vi "niScope Multi Fetch WDT_noERROR.vi"(6 "numSamples":i32=-1, 7 "timestamp Type":T1=1 caption="timestamp type" items=["relative", "absolute"], 8 "error in":errorcluster, 9 "timeout":dbl=5.0 format="%.2f", 10 "channels":string="0", 11 "instrument handle":refnum<k15>) -> (0 "error out":errorcluster, 1 "wfm":waveform(dbl)[](array[waveform]), 2 "wfm info":T2(array[cluster]) {"reserved2" format="%.2f"; "reserved1" format="%.2f"; "offset" format="%^.3e"; "gain" format="%^.3e"; "xIncrement" format="%^.3e"; "relativeInitialX" format="%^.3e"; "absoluteInitialX" format="%^.3e"}, 3 "instrument handle out":refnum<k15>)   [LabVIEW 2010]
uses:
  <instrlib>/niScope/Controls/niScope timestamp type.ctl
  niScope_32.dll
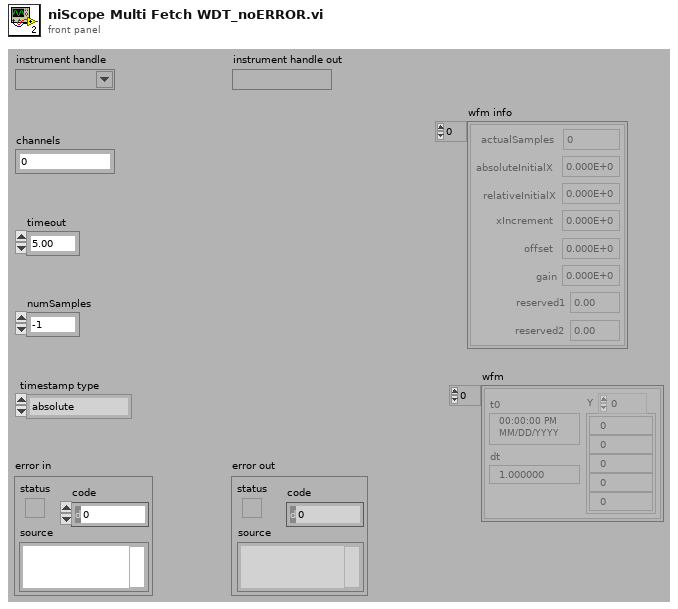
[diagram p1: front panel]
types:
  T1 = typedef "niScope timestamp type.ctl" = i32
  T2 = cluster{"actualSamples":i32, "absoluteInitialX":dbl, "relativeInitialX":dbl, "xIncrement":dbl, "offset":dbl, "gain":dbl, "reserved1":dbl, "reserved2":dbl}[]
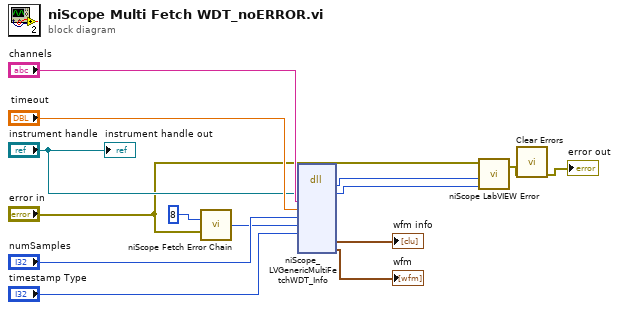
[diagram p0: block diagram]
diagram:
  n1 = call <instrlib>:"niScope Fetch Error Chain.vi"("dataType in"=8 ("dataType"), "error in"="error in") -> ("dataType"=w6:i32)  [unwired: 13 in]
  n2 = dll-call lib="niScope_*.*" fn="niScope_LVGenericMultiFetchWDT_Info"("instrument handle"="instrument handle", "channelList"="channels", "timeout"="timeout", "numSamples"="numSamples", "dataType"=w6, "timestampType"="timestamp Type") -> ("status"=w11:i32, "instrument handle"=w10:u32, "wfm info"=→"wfm info":T2, "wfm"=→"wfm":waveform(dbl)[])  [unwired: 10 in, 2 out]
  n3 = call <instrlib>:"niScope LabVIEW Error.vi"("instrument handle"=w10, "niScope error code (0)"=w11, "error in (no error)"="error in") -> ("error out"=w1:errorcluster)  [unwired: 2 in]
  n4 = call <vilib>:"Clear Errors.vi"("error in (no error)"=w1) -> ("error out"=→"error out":errorcluster)  [unwired: 6 in]
  "instrument handle out" <- "instrument handle"
